vi "Write Text.vi"(8 "error in (no error)":errorcluster, 9 "Text":string, 10 "Header":string, 11 "Log File Ref":refnum<data-value>) -> (0 "error out":errorcluster, 3 "Log File Ref":refnum<data-value>)   [LabVIEW 2014, in "Log File.lvclass"]
uses:
  Log File.lvclass
  Log File.lvclass/Log File.ctl
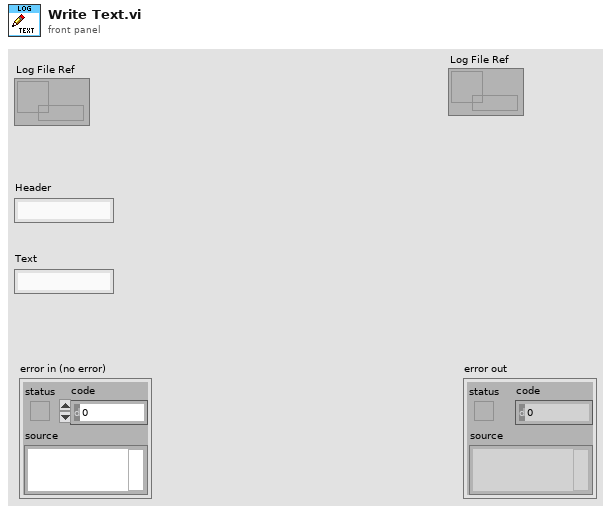
[diagram p1: front panel]
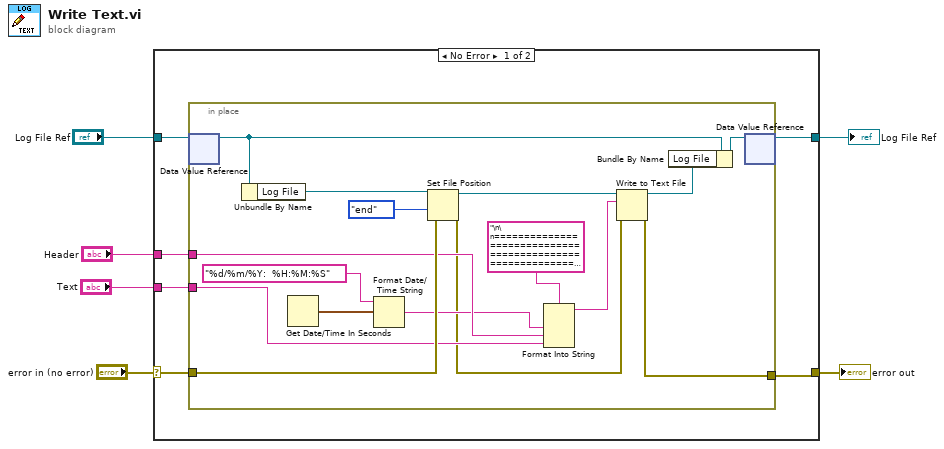
[diagram p0: block diagram]
diagram:
  n1 = case shown="No Error" "error in (no error)" {
    selector: "error in (no error)" -> [w11 w30]
    tunnel: [w8 w30] -> w5
    tunnel: "Log File Ref" -> [w12 w29]
    tunnel: "Header" -> [w10 _]
    tunnel: "Text" -> [w9 _]
    tunnel: [w7 w29] -> w1
    frame No Error {
      n2 = in-place {
        in-place-border: w11 -> [w26]
        in-place-border: w10 -> [w23]
        in-place-border: w9 -> [w22]
        in-place-border: [w17] -> w8
        n3 = in-place-dvr #1(w12) -> (w16:refnum<class "Log File.lvclass">)  [unwired: 1 out]
        n4 = Unbundle By Name(w16) -> ("Log File"=w27:refnum<file>)
        n5 = Get Date/Time In Seconds() -> (seconds since 1Jan1904=w21:timestamp)
        n6 = Format Date/Time String(time format string (%c)="%d/%m/%Y:  %H:%M:%S", seconds (now)=w21) -> (date/time string=w19:string)  [unwired: 1 in]
        n7 = Set File Position(refnum=w27, from (0:start)=enum16{"start", "end", "current"}."end", error in=w26) -> (refnum out=w25:refnum<file>, error out=w18:errorcluster)  [unwired: 1 in]
        n8 = Format Into String(format string="\n\n========================================================================================================\n%s ---- %s\n\n%s", w19, w23, w22) -> (resulting string=w24:string)  [unwired: 2 in, 1 out]
        n9 = Write to Text File(file (use dialog)=w25, text=w24, error in=w18) -> (refnum out=w15:refnum<file>, error out=w17:errorcluster)  [unwired: 1 in, 1 out]
        n10 = Bundle By Name(cluster=w16, "Log File"=w15) -> (w14:refnum<class "Log File.lvclass">)
        n11 = in-place-dvr #1(w14) -> (w7:refnum<data-value>)  [unwired: 1 out]
      }
    }
    frame Error {
    }
  }
  "error out" <- w5
  "Log File Ref" <- w1
